vi "AlliGator Last Gate Loading.vi"(0 "Dataset Images 1 in":T1, 1 "Gates across boundaries?":bool, 2 "Split Index":u32, 5 "Dataset Images 2 in":T1, 7 "Current Gate":i32, 9 "VI in":refnum<vi>, 11 "error in (no error)":errorcluster) -> (4 "Dataset Images 1 out":T1, 6 "Dataset Images 2 out":T1, 10 "# Disposed Images":i32, 15 "error out":errorcluster)   [LabVIEW 2021, in "AlliGator Files.lvlib"]
doc: "Last gate image loading actions and house-keeping."
uses:
  AlliGator Files.lvlib
  Internal Variables/AlliGator Gate Image Set.ctl
  <vilib>/vision/Image Controls.llb/IMAQ Image.ctl
  HDF5/AlliGator FLI Image Stack Action.ctl
  HDF5/AlliGator HDF5.lvlib
  Image/Image.lvlib
  Internal Variables/AlliGator Internal Variables.lvlib
panel:
  # "see the AlliGator License on the block diagram (Ctrl+E or Window:Show Block Diagram)"
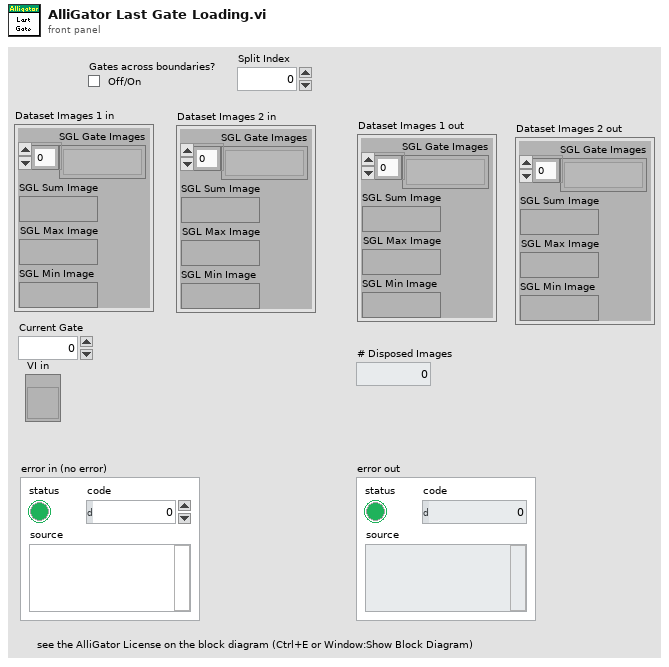
[diagram p1: front panel]
types:
  T1 = typedef "AlliGator Internal Variables.lvlib/AlliGator Gate Image Set.ctl" = cluster{"SGL Gate Images":T2[], "SGL Sum Image":T2, "SGL Max Image":T2, "SGL Min Image":T2}
  T2 = typedef "IMAQ Image.ctl" = refnum<image>
  T3 = typedef "AlliGator HDF5.lvlib/AlliGator FLI Image Stack Action.ctl" = enum16{"Init", "Get Image", "Close"}
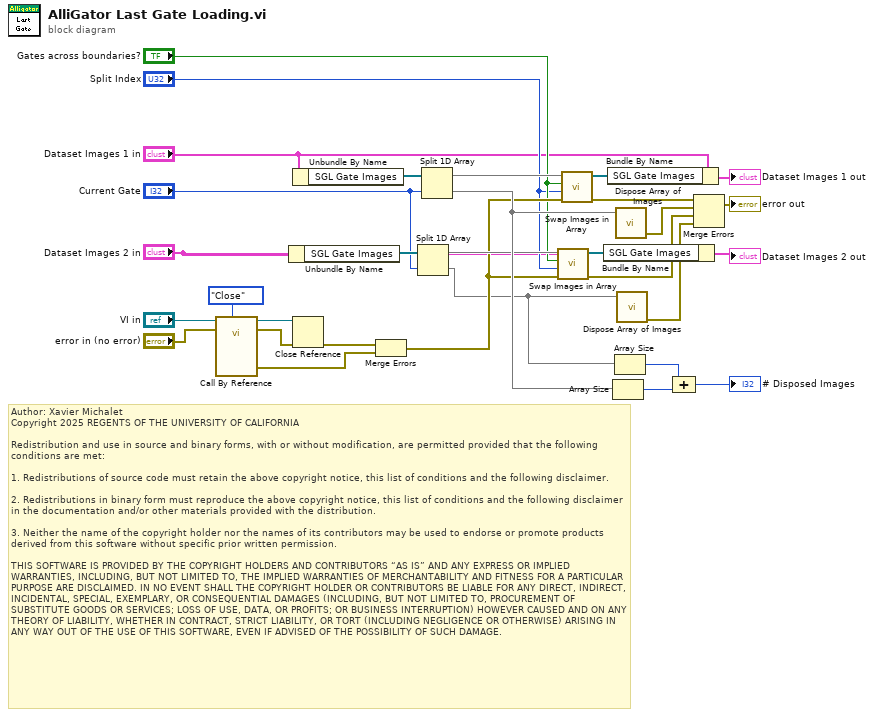
[diagram p0: block diagram]
diagram:
  # "Author: Xavier Michalet\nCopyright 2025 REGENTS OF THE UNIVERSITY OF CALIFORNIA\n\nRedistribution and use in source and binary forms, with or without modification, are permitted provided that the following conditions are met:\n\n1. Redistributions of source code must retain the above copyright notice, this list of conditions and the following disclaimer.\n\n2. Redistributions in binary form must reproduce the above copyright notice, this list of conditions and the following disclaimer in the documentation and/or other materials provided with the distribution.\n\n3. Neither the name of the copyright holder nor the names of its contributors may be used to endorse or promote products derived from this software without specific prior written permission.\n\nTHIS SOFTWARE IS PROVIDED BY THE COPYRIGHT HOLDERS AND CONTRIBUTORS “AS IS” AND ANY EXPRESS OR IMPLIED WARRANTIES, INCLUDING, BUT NOT LIMITED TO, THE IMPLIED WARRANTIES OF MERCHANTABILITY AND FITNESS FOR A PARTICULAR PURPOSE ARE DISCLAIMED. IN NO EVENT SHALL THE COPYRIGHT HOLDER OR CONTRIBUTORS BE LIABLE FOR ANY DIRECT, INDIRECT, INCIDENTAL, SPECIAL, EXEMPLARY, OR CONSEQUENTIAL DAMAGES (INCLUDING, BUT NOT LIMITED TO, PROCUREMENT OF SUBSTITUTE GOODS OR SERVICES; LOSS OF USE, DATA, OR PROFITS; OR BUSINESS INTERRUPTION) HOWEVER CAUSED AND ON ANY THEORY OF LIABILITY, WHETHER IN CONTRACT, STRICT LIABILITY, OR TORT (INCLUDING NEGLIGENCE OR OTHERWISE) ARISING IN ANY WAY OUT OF THE USE OF THIS SOFTWARE, EVEN IF ADVISED OF THE POSSIBILITY OF SUCH DAMAGE."
  n1 = call-by-ref "?"(reference="VI in", error in="error in (no error)", "Action"=AlliGator_FLI_Image_Stack_Action."Close") -> (reference out=w19:refnum<vi>, error out=w20:errorcluster, 0:"error out"=w23:errorcluster)  [unwired: 8 in, 2 out]
  n2 = Unbundle By Name("Dataset Images 2 in") -> ("SGL Gate Images"=w13:T2[])
  n3 = Unbundle By Name("Dataset Images 1 in") -> ("SGL Gate Images"=w31:T2[])
  n4 = Close Reference(reference=w19, error in (no error)=w20) -> (error out=w16:errorcluster)
  n5 = Merge Errors(w16, w23) -> (w11:errorcluster)
  n6 = Split 1D Array(array=w13, index="Current Gate") -> (first subarray=w15:T2[], second subarray=w10:T2[])
  n7 = Split 1D Array(array=w31, index="Current Gate") -> (first subarray=w29:T2[], second subarray=w27:T2[])
  n8 = call "Swap Images in Array.vi"("Error In"=w11, "Split Index"="Split Index", "Swap Images?"="Gates across boundaries?", "Image Array in"=w15) -> ("Error Out"=w1:errorcluster, "Image Array out"=w14:T2[])  [unwired: 6 in]
  n9 = call "Swap Images in Array.vi"("Error In"=w11, "Split Index"="Split Index", "Swap Images?"="Gates across boundaries?", "Image Array in"=w29) -> ("Error Out"=w28:errorcluster, "Image Array out"=w30:T2[])  [unwired: 6 in]
  n10 = Bundle By Name(cluster="Dataset Images 2 in", "SGL Gate Images"=w14) -> (→"Dataset Images 2 out":T1)
  n11 = Bundle By Name(cluster="Dataset Images 1 in", "SGL Gate Images"=w30) -> (→"Dataset Images 1 out":T1)
  n12 = Array Size(array=w27) -> (size(s)=w17:i32)
  n13 = Array Size(array=w10) -> (size(s)=w7:i32)
  n14 = call "Dispose Array of Images.vi"("Array of Images"=w27) -> ("error out"=w26:errorcluster)  [unwired: 8 in]
  n15 = call "Dispose Array of Images.vi"("Array of Images"=w10) -> ("error out"=w9:errorcluster)  [unwired: 8 in]
  n16 = Compound Arithmetic op=ADD(w7, w17) -> (→"# Disposed Images":i32)
  n17 = Merge Errors(w28, w26, w1, w9) -> (→"error out":errorcluster)
